vi "Write Data.vi"(8 "error in (no error)":errorcluster, 10 "Data":string, 11 "WebSocket Data Handler Msg in":refnum<class "WebSocket Connection Handler Msg.lvclass">) -> (0 "error out":errorcluster, 3 "WebSocket Data Handler Msg out":refnum<class "WebSocket Connection Handler Msg.lvclass">)   [LabVIEW 2016, in "WebSocket Actors.lvlib" / "WebSocket Connection Handler Msg.lvclass"]
uses:
  WebSocket Connection Handler Msg.lvclass
  WebSocket Connection Handler Msg.lvclass/WebSocket Connection Handler Msg.ctl
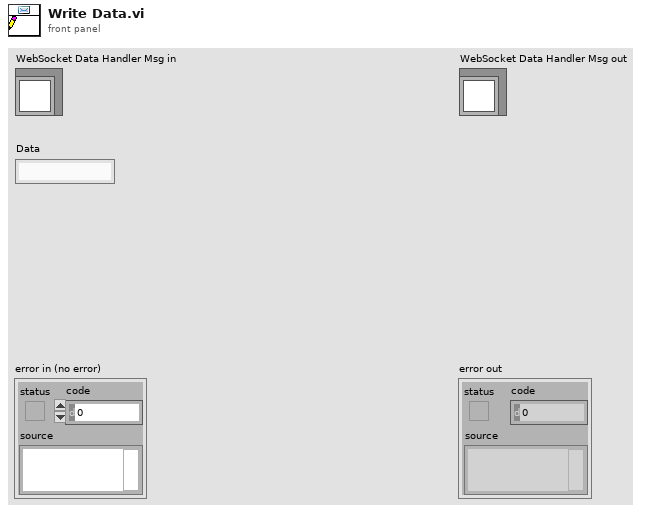
[diagram p1: front panel]
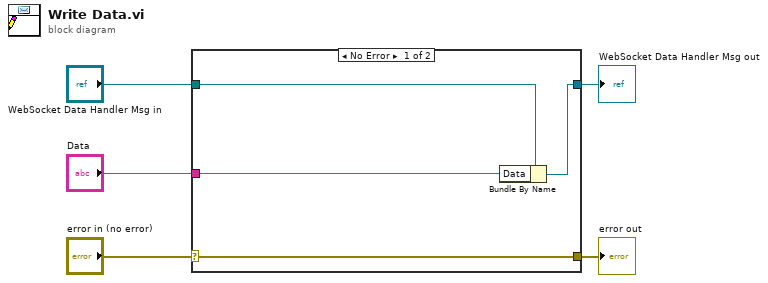
[diagram p0: block diagram]
diagram:
  n1 = case shown="No Error" "error in (no error)" {
    selector: "error in (no error)" -> [w9 w10]
    tunnel: [w9 w10] -> w4
    tunnel: [w7 w11] -> w2
    tunnel: "WebSocket Data Handler Msg in" -> [w8 w11]
    tunnel: "Data" -> [w6 _]
    frame No Error {
      n2 = Bundle By Name(cluster=w8, "Data"=w6) -> (w7:refnum<class "WebSocket Connection Handler Msg.lvclass">)
    }
    frame Error {
    }
  }
  "error out" <- w4
  "WebSocket Data Handler Msg out" <- w2
